vi "GenerateUserEvent.vi"(8 "error in (no error)":errorcluster, 10 "anything":cluster{"Boolean":bool}, 11 "Event Actions":T1(ring)=enum."Generate Event") -> (0 "error out":errorcluster, 3 "UserEvent":refnum<user-event>)   [LabVIEW 2013]
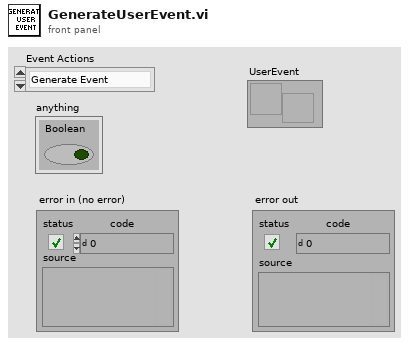
[diagram p1: front panel]
types:
  T1 = enum16{"Create Event", "Generate Event", "Destroy Event"}
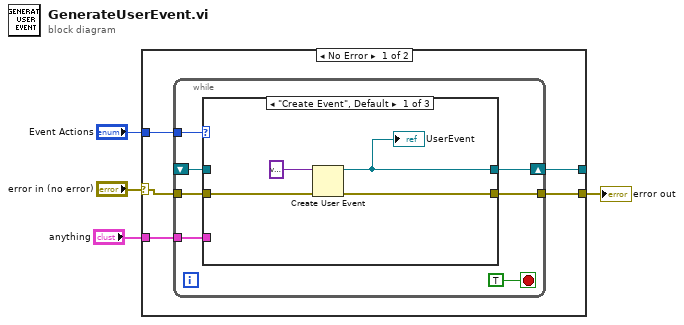
[diagram p0: block diagram]
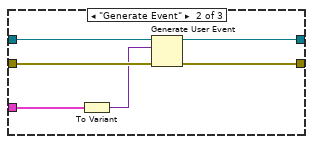
[diagram p2: hidden frame]
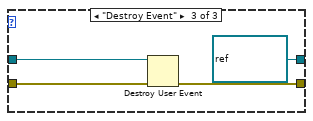
[diagram p3: hidden frame]
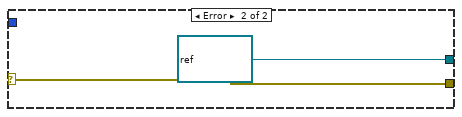
[diagram p4: hidden frame]
diagram:
  n1 = case shown="No Error" "error in (no error)" {
    selector: "error in (no error)" -> [w8 w32]
    tunnel: "Event Actions" -> [w9 _]
    tunnel: [w7 w32] -> w2
    tunnel: "anything" -> [w6 _]
    tunnel: [w5 refnum<user-event> refnum ("Variant")] -> _
    frame No Error {
      n2 = while {
        tunnel: w9 -> [w16]
        tunnel: [w14] -> w7
        shift-right: [w15] -> w5
        shift-left: _ -> [w13]
        tunnel: w8 -> [w12]
        tunnel: w6 -> [w11]
        stop <- TRUE stop-if-true
        n3 = case shown="\"Create Event\", Default" w16 {
          tunnel: [w17 w25 refnum<user-event> refnum ("Variant")] -> w15
          tunnel: [w20 w26 w30] -> w14
          tunnel: w13 -> [_ w24 w28]
          tunnel: w12 -> [w19 w23 w29]
          tunnel: w11 -> [_ w21 _]
          frame "Create Event", Default {
            n4 = Create User Event(user event datatype=variant ("variant"), error in=w19) -> (user event=w17:refnum<user-event>, error out=w20:errorcluster)
            "UserEvent" <- w17
          }
          frame "Generate Event" {
            n5 = To Variant(anything=w21) -> (Variant=w22:variant)
            n6 = Generate User Event(user event=w24, event data cluster=w22, error in=w23) -> (user event out=w25:refnum<user-event>, error out=w26:errorcluster)  [unwired: 1 in]
          }
          frame "Destroy Event" {
            n7 = Destroy User Event(user event=w28, error in=w29) -> (error out=w30:errorcluster)
          }
        }
      }
    }
    frame Error {
    }
  }
  "error out" <- w2
